vi "Periodic Tasks.vi"(8 "error in (no error)":errorcluster) -> ()   [LabVIEW 2017]
doc: "This VI runs in parallel to other tasks. It can contain as many user-defined periodic loops as you need. These can carry out PID or other sorts of timed response."
uses:
  Robot Global Data.vi
  <vilib>/Rock Robotics/WPI/Utilities/WPI_GetSetVariantRefNum.vi
  <vilib>/addons/control/pid/pid.llb/PID (DBL).vi
  <vilib>/Rock Robotics/Network Tables/NT Read Number.vi
  <vilib>/Rock Robotics/WPI/RobotDrive/WPI_RobotDriveArcadeDrive_Standard(NoSaturation).vi
  <vilib>/Rock Robotics/Network Tables/NT Write Number.vi
  <vilib>/addons/control/pid/NI_PID_pid.lvlib
  <vilib>/Analysis/NI_AALPro.lvlib
  <vilib>/Analysis/coordinate.llb/2D Cartesian Coordinate Shift (Scalar).vi
  <vilib>/Rock Robotics/Network Tables/NT Read String.vi
  <vilib>/Analysis/coordinate.llb/2D Cartesian Coordinate Shift (Array).vi
  <vilib>/Analysis/coordinate.llb/2D Cartesian Coordinate Rotation (Scalar).vi
panel:
  out "Waveform Chart":dbl(graph)
  out "CDF Arm Down":bool
  out "error out (no error)":errorcluster
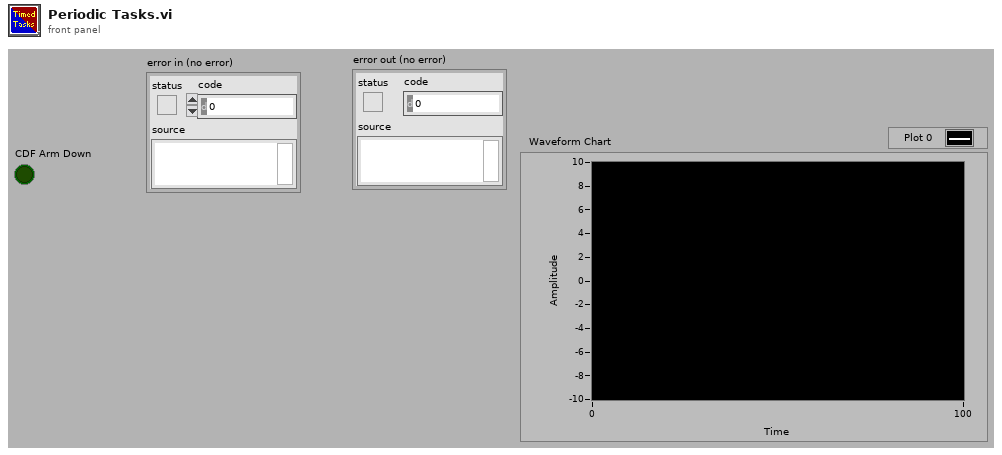
[diagram p1: front panel]
types:
  T1 = cluster{"theta":dbl, "x":dbl, "y":dbl, "xServo":dbl, "yServo":dbl}
  T2 = typedef "WPI_PotentiometerDevRef.ctl" = cluster{"DevStatus":errorcluster, "Analog Channel":T3, "Invert Output":bool}
  T3 = typedef "FPGA_AIChannel.ctl" = enum8{"AI 0", "AI 1", "AI 2", "AI 3", "AI MXP 0", "AI MXP 1", "AI MXP 2", "AI MXP 3", "Invalid"}
  T4 = typedef "WPI_ServoDeviceRef.ctl" = cluster{"DeviceStatus":errorcluster, "PWM Channel":T5, "DeadBand":T6}
  T5 = typedef "FPGA_DIOPWMChannel.ctl" = enum8{"PWM 0", "PWM 1", "PWM 2", "PWM 3", "PWM 4", "PWM 5", "PWM 6", "PWM 7", "PWM 8", "PWM 9", "PWM MXP 0", "PWM MXP 1", "PWM MXP 2", "PWM MXP 3", "PWM MXP 4", "PWM MXP 5", "PWM MXP 6", "PWM MXP 7", "PWM MXP 8", "PWM MXP 9", "Invalid"}
  T6 = typedef "WPI_PWMDeadband.ctl" = cluster{"Name":string, "maxPositivePwm":i32, "minPositivePwm":i32, "centerPwm":i32, "maxNegativePwm":i32, "minNegativePwm":i32, "angularRange":u16}
  T7 = typedef "WPI_GyroDevRef.ctl" = cluster{"DevStatus":errorcluster, "Analog Channel":T3, "Gain (VoltsPerDegree/Second)":dbl, "Gyro Type":enum16{"Analog", "XRS450"}, "Handle":i32, "SPI Bus":T8, "Device Found":bool, "Sample Rate":dbl, "Calibrate On Open":bool, "Offset":dbl}
  T8 = typedef "spi_bus.ctl" = enum16{"SPI On-Board, CS0", "SPI On-Board, CS1", "SPI On-Board, CS2", "SPI On-Board, CS3", "SPI MXP", "Invalid"}
  T9 = cluster{"theta":dbl, "x":dbl, "y":dbl, "xServo":dbl, "yServo":dbl}[]
  T10 = typedef "WPI_RobotDriveDevRef.ctl" = cluster{"DevStatus":errorcluster, "Motors[]":T11[], "Square Inputs":bool, "Max Output":dbl}
  T11 = typedef "WPI_MotorControlDeviceRef.ctl" = cluster{"DeviceStatus":errorcluster, "Type":T12, "PWM":cluster{"PWM Channel":T5, "DeadBand":T6}, "CAN":cluster{"Device Number":u8, "SetOutput VI Ref":variant, "GetOutput VI Ref":variant, "Enable VI Ref":variant, "Disable VI Ref":variant, "Data":variant}, "Invert":bool, "DIO PWM":cluster{"PWM \"Enable\" Channel":T5, "DIOChannel":T13, "PWM Rate":dbl}}
  T12 = typedef "WPI_MotorControlType.ctl" = enum16{"PWM", "CAN", "DIO PWM"}
  T13 = typedef "FPGA_DIOChannel.ctl" = enum8{"DIO 0", "DIO 1", "DIO 2", "DIO 3", "DIO 4", "DIO 5", "DIO 6", "DIO 7", "DIO 8", "DIO 9", "DIO MXP 0", "DIO MXP 1", "DIO MXP 2", "DIO MXP 3", "DIO MXP 4", "DIO MXP 5", "DIO MXP 6", "DIO MXP 7", "DIO MXP 8", "DIO MXP 9", "DIO MXP 10", "DIO MXP 11", "DIO MXP 12", "DIO MXP 13", "DIO MXP 14", "DIO MXP 15", "SPI Port CS1", "SPI Port CS2", "SPI Port CS3", "SPI Port MISO", "SPI Port MOSI", "Invalid"}
  T14 = cluster{"proportional gain (Kc)":dbl, "integral time (Ti, min)":dbl, "derivative time (Td, min)":dbl}
  T15 = typedef "WPI_AccelerometerDevRef.ctl" = cluster{"DevStatus":errorcluster, "Scaling":T16, "Analog Channels":T17, "I2C Bus":T18, "SPI Bus":T8, "Accel Range":T19, "ADXL Axes":T20, "Handle":i32, "Device Address":u8, "Accel Type":enum16{"Analog", "ADXL345 I2C", "ADXL345 SPI", "Internal", "ADXL362 SPI"}}
  T16 = typedef "WPI_AccelerometerScaling.ctl" = cluster{"Gain (VoltsPerG)":dbl, "Center Voltage":dbl}
  T17 = typedef "WPI_AccelerometerAnalogChannels.ctl" = cluster{"X-Axis":T3, "Y-Axis":T3, "Z-Axis":T3}
  T18 = typedef "i2c_bus.ctl" = enum16{"I2C On-Board", "I2C MXP", "Invalid"}
  T19 = typedef "ADXL345 Range.ctl" = u8
  T20 = typedef "WPI_AccelerometerADXL345 Axes.ctl" = cluster{"X-Axis":bool, "Y-Axis":bool, "Z-Axis":bool}
  T21 = cluster{"X-Axis":dbl, "Y-Axis":dbl, "Z-Axis":dbl}
  T22 = enum16{"open", "replace", "create", "open or create", "replace or create", "replace or create with confirmation"}
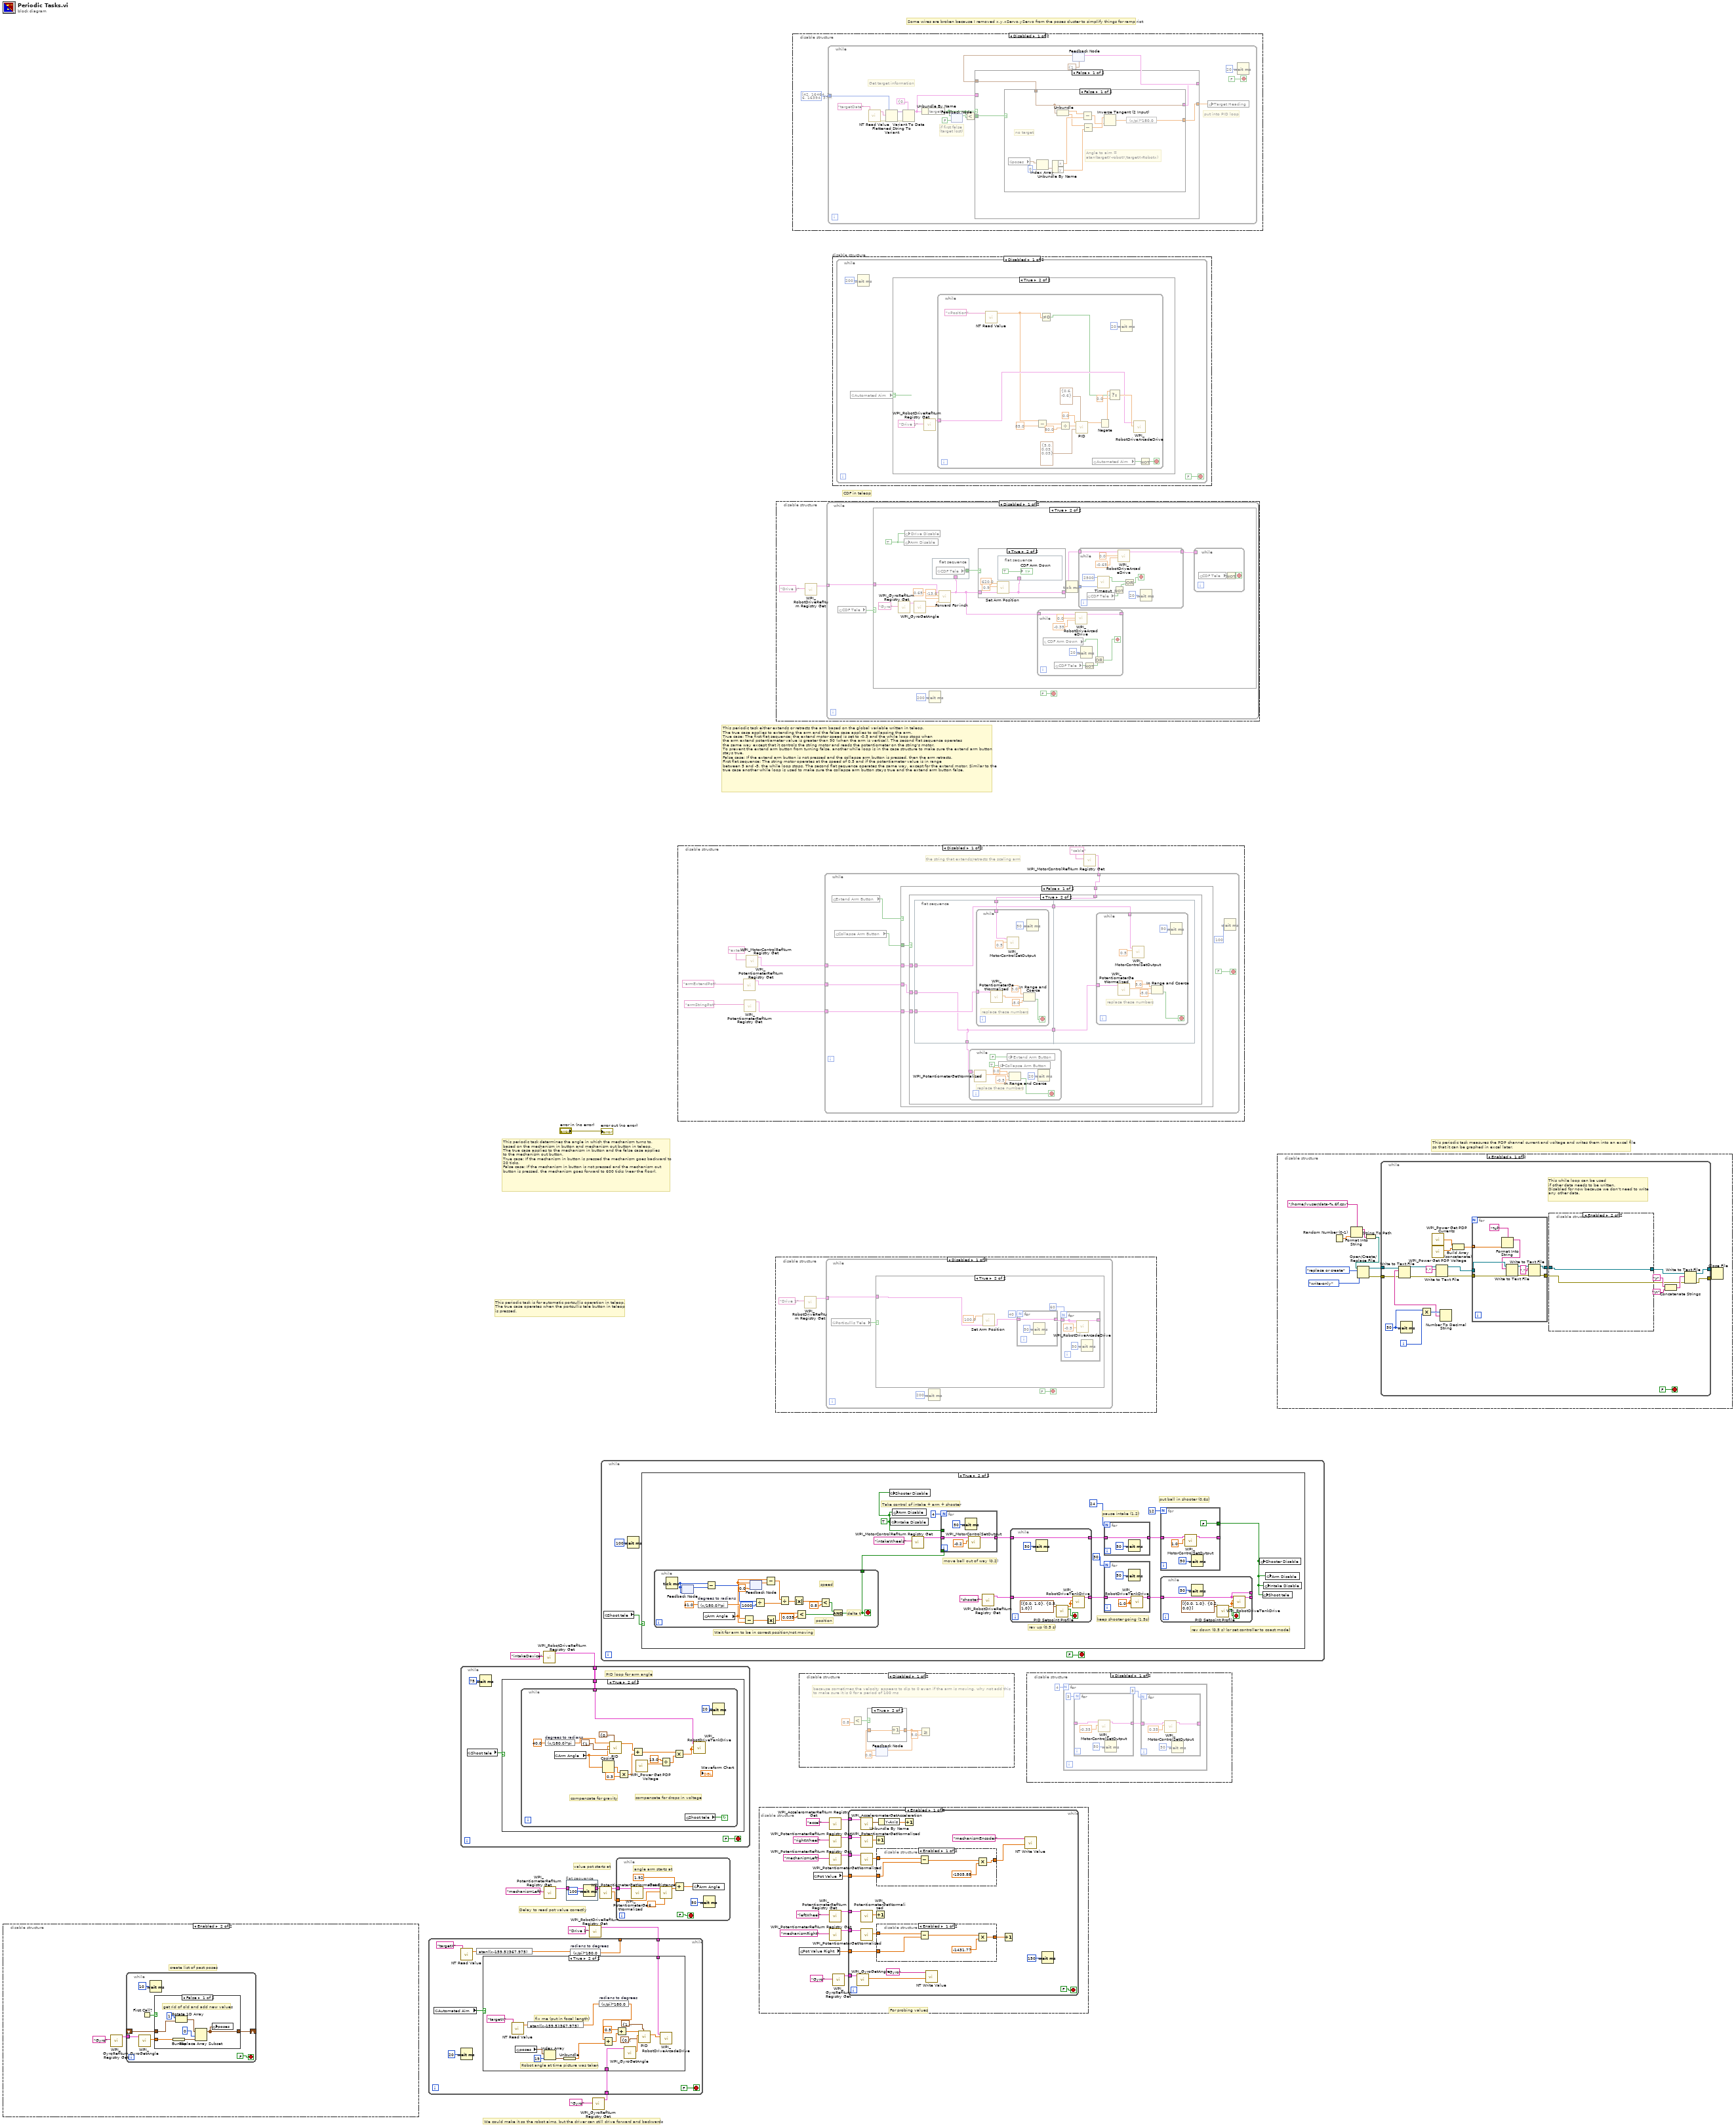
[diagram p0: block diagram]
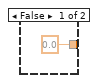
[diagram p4: hidden frame]
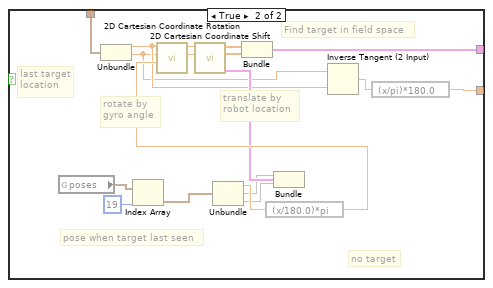
[diagram p8: hidden frame]
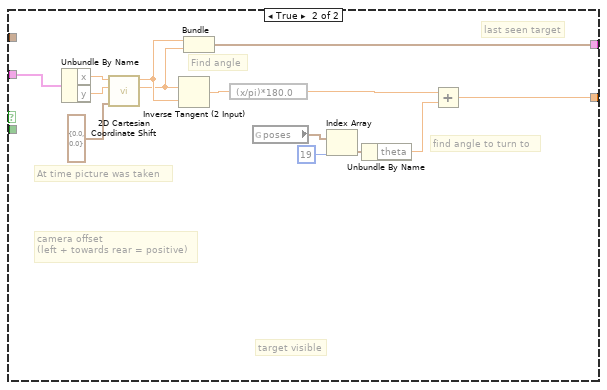
[diagram p9: hidden frame]
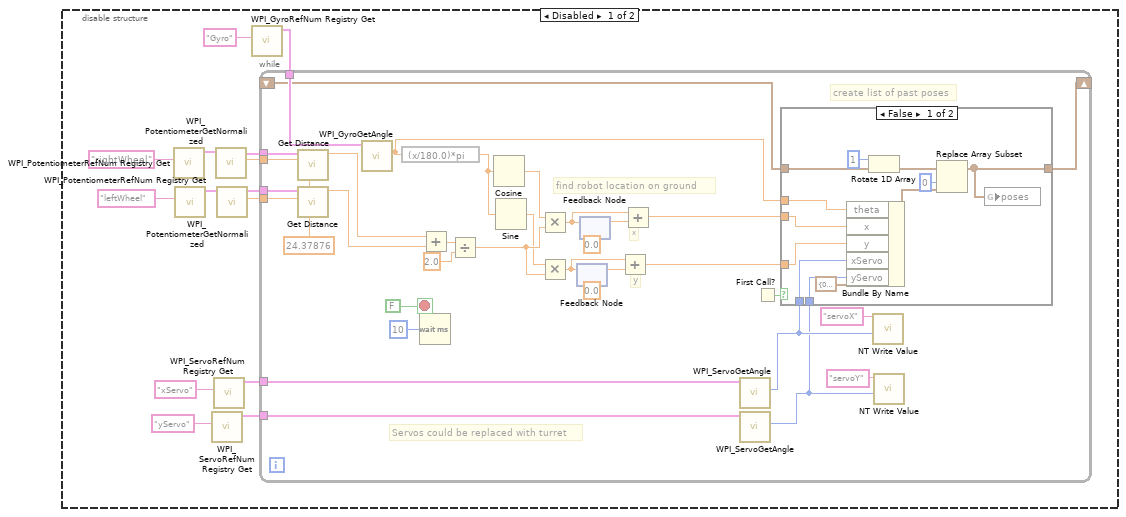
[diagram p11: hidden frame]
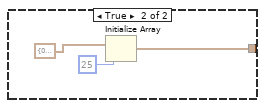
[diagram p12: hidden frame]
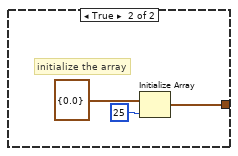
[diagram p13: hidden frame]
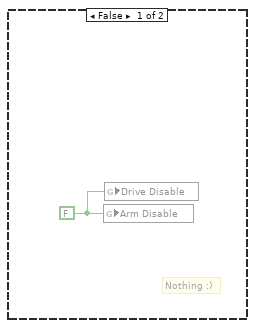
[diagram p16: hidden frame]
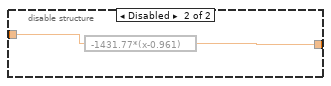
[diagram p19: hidden frame]
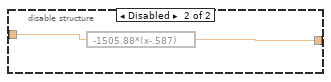
[diagram p20: hidden frame]
diagram:
  # "We could make it so the robot aims, but the driver can still drive forward and backwards"
  # "Delay to read pot value correctly"
  # "Some wires are broken because I removed x,y,xServo,yServo from the poses cluster to simplify things for ramp riot"
  # "value pot starts at"
  # "CDF in teleop"
  # "This periodic task either extends or retracts the arm based on the global variable written in teleop.\nThe true case applies to extending the arm and the false case applies to collapsing the arm. \nTrue case: The first flat sequence: the extend motor speed is set to -0.5 and the while loop stops when\nthe arm extend potentiameter value is greater than 90 (when the arm is vertical). The second flat sequence operates\nthe same way except that it controls the string motor and reads the potentiometer on the string's motor. \nTo prevent the extend arm button from turning false, another while loop is in the case structure to make sure the extend arm button \nstays true. \nFalse case: If the extend arm button is not pressed and the collapse arm button is pressed, then the arm retracts.\nFirst flat sequence: The string motor operates at the speed of 0.5 and if the potentiameter value is in range \nbetween 5 and -5, the while loop stops. The second flat sequence operates the same way, except for the extend motor. Similar to the \ntrue case another while loop is used to make sure the collapse arm button stays true and the extend arm button false."
  # "This periodic task measures the PDP channel current and voltage and writes them into an excel file \nso that it can be graphed in excel later."
  # "This periodic task is for automatic portcullis operation in teleop. \nThe true case operates when the portcullis tele button in teleop \nis pressed."
  # "This periodic task determines the angle in which the mechanism turns to, \nbased on the mechanism in button and mechanism out button in teleop.\nThe true case applies to the mechanism in button and the false case applies\nto the mechanism out button. \nTrue case: If the mechanism in button is pressed the mechanism goes backward to\n20 ticks. \nFalse case: If the mechanism in button is not pressed and the mechanism out\nbutton is pressed, the mechanism goes forward to 600 ticks (near the floor)."
  n1 = disable-structure shown="Enabled" {
    frame Disabled {
      n2 = call <vilib>:"WPI_PotentiometerRefNum Registry Get.vi"("refnum name"="rightWheel") -> ("PotDevRef"=w26:T2)  [unwired: 9 in, 1 out]
      n3 = call <vilib>:"WPI_PotentiometerRefNum Registry Get.vi"("refnum name"="leftWheel") -> ("PotDevRef"=w24:T2)  [unwired: 9 in, 1 out]
      n4 = call <vilib>:"WPI_ServoRefNum Registry Get.vi"("refnum name"="yServo") -> ("ServoDeviceRef"=w13:T4)  [unwired: 9 in, 1 out]
      n5 = call <vilib>:"WPI_ServoRefNum Registry Get.vi"("refnum name"="xServo") -> ("ServoDeviceRef"=w14:T4)  [unwired: 9 in, 1 out]
      n6 = call <vilib>:"WPI_PotentiometerGetNormalized.vi"("PotDevRef"=w26) -> ("Normalized Value"=w18:dbl, "PotDevRef"=w21:T2)  [unwired: 8 in, 1 out]
      n7 = call <vilib>:"WPI_PotentiometerGetNormalized.vi"("PotDevRef"=w24) -> ("Normalized Value"=w19:dbl, "PotDevRef"=w20:T2)  [unwired: 8 in, 1 out]
      n8 = call <vilib>:"WPI_GyroRefNum Registry Get.vi"("refnum name"="Gyro") -> ("GyroDevRef"=w17:T7)  [unwired: 9 in, 1 out]
      n9 = while {
        tunnel: w21 -> [w59]
        tunnel: w20 -> [w58]
        tunnel: w19 -> [w57]
        tunnel: w18 -> [w56]
        tunnel: w17 -> [w39]
        shift-right: [w35] -> _
        shift-left: _ -> [w34]
        tunnel: w14 -> [w30]
        tunnel: w13 -> [w29]
        stop <- FALSE stop-if-true
        w55 = 24.37876 ("distance/rotation")
        # "Servos could be replaced with turret"
        # "create list of past poses"
        # "find robot location on ground"
        # "y"
        # "x"
        n10 = call "Get Distance.vi"("distance/rotation"=w55, "Starting value"=w56, "PotDevRef"=w59) -> ("Distance"=w41:dbl)  [unwired: 8 in]
        n11 = call "Get Distance.vi"("distance/rotation"=w55, "Starting value"=w57, "PotDevRef"=w58) -> ("Distance"=w40:dbl)  [unwired: 8 in]
        n12 = call <vilib>:"WPI_GyroGetAngle.vi"("GyroDevRef"=w39) -> ("Angle"=w33:dbl)  [unwired: 6 in, 4 out]
        n13 = expression code="(x/180.0)*pi" ("degrees to radians")(w33) -> (w50:dbl)
        n14 = Wait (ms)(milliseconds to wait=u32 10) -> ()  [unwired: 1 out]
        n15 = Add(x=w41, y=w40) -> (x+y=w53:dbl)
        n16 = Divide(x=w53, y=2.0) -> (x/y=w49:dbl)
        n17 = Cosine(x=w50) -> (cos(x)=w51:dbl)
        n18 = Sine(x=w50) -> (sin(x)=w48:dbl)
        n19 = Multiply(x=w51, y=w49) -> (x*y=w46:dbl)
        n20 = Multiply(x=w48, y=w49) -> (x*y=w42:dbl)
        n21 = feedback #1(0.0) -> (w43:dbl)
        n22 = feedback-in #1(w42) -> ()
        n23 = feedback #2(0.0) -> (w47:dbl)
        n24 = feedback-in #2(w46) -> ()
        n25 = Add(x=w42, y=w43) -> (x+y=w32:dbl)
        n26 = Add(x=w46, y=w47) -> (x+y=w31:dbl)
        n27 = call <vilib>:"WPI_ServoGetAngle.vi"("ServoDeviceRef"=w30) -> ("Angle"=w28:u16)  [unwired: 7 in, 2 out]
        n28 = call <vilib>:"WPI_ServoGetAngle.vi"("ServoDeviceRef"=w29) -> ("Angle"=w27:u16)  [unwired: 7 in, 2 out]
        n29 = First Call?() -> (First Call?: T/F=w38:bool)
        n30 = case shown="False" w38 {
          tunnel: [w61 w74] -> w35
          tunnel: w34 -> [w72 _]
          tunnel: w33 -> [w68 _]
          tunnel: w31 -> [w64 _]
          tunnel: w32 -> [w65 _]
          tunnel: w28 -> [w63 _]
          tunnel: w27 -> [w62 _]
          frame False {
            n31 = Bundle By Name(cluster=T1 {"theta"=0.0, "x"=0.0, "y"=0.0, "xServo"=0.0, "yServo"=0.0}, "theta"=w68, "x"=w64, "y"=w65, "xServo"=w63, "yServo"=w62) -> (w66:T1)
            n32 = Rotate 1D Array(1:w72, 2:1 ("n")) -> (0:w70:T9)
            n33 = Replace Array Subset(array=w70, new element=w66, index=0) -> (w61:T9)
            n34 = global write "Robot Global Data.vi" "poses"(w61) -> ()
          }
          frame True {
            n35 = Initialize Array(T1 {"theta"=0.0, "x"=0.0, "y"=0.0, "xServo"=0.0, "yServo"=0.0}, 25 ("dimension size")) -> (w74:T9)
          }
        }
        n36 = call-poly <vilib>:"NT Write Value.vi"("Numeric"=w28, "Name"="servoX") -> ()  [unwired: 9 in, 1 out]
        n37 = call-poly <vilib>:"NT Write Value.vi"("Numeric"=w27, "Name"="servoY") -> ()  [unwired: 9 in, 1 out]
      }
    }
    frame Enabled {
      # "create list of past poses"
      n38 = call <vilib>:"WPI_GyroRefNum Registry Get.vi"("refnum name"="Gyro") -> ("GyroDevRef"=w76:T7)  [unwired: 9 in, 1 out]
      n39 = while {
        tunnel: w76 -> [w82]
        shift-right: [w80] -> _
        shift-left: _ -> [w79]
        stop <- FALSE stop-if-true
        n40 = call <vilib>:"WPI_GyroGetAngle.vi"("GyroDevRef"=w82) -> ("Angle"=w78:dbl)  [unwired: 6 in, 4 out]
        n41 = First Call?() -> (First Call?: T/F=w81:bool)
        n42 = Wait (ms)(milliseconds to wait=u32 10) -> ()  [unwired: 1 out]
        n43 = case shown="False" w81 {
          tunnel: [w87 w93] -> w80
          tunnel: w79 -> [w91 _]
          tunnel: w78 -> [w86 _]
          frame False {
            # "get rid of old and add new values"
            n44 = Bundle("Angle"=w86) -> (w85:cluster{"Angle":dbl})  [unwired: 1 in]
            n45 = Rotate 1D Array(1:w91, 2:1 ("n")) -> (0:w89:cluster{"theta":dbl}[])
            n46 = Replace Array Subset(array=w89, new element=w85, index=0) -> (w87:cluster{"theta":dbl}[])
            n47 = global write "Robot Global Data.vi" "poses"(w87) -> ()
          }
          frame True {
            # "initialize the array"
            n48 = Initialize Array(cluster{"theta":dbl} {"theta"=0.0}, 25 ("dimension size")) -> (w93:cluster{"theta":dbl}[])
          }
        }
      }
    }
  }
  n49 = call <vilib>:"WPI_RobotDriveRefNum Registry Get.vi"("refnum name"="intakeDevice") -> ("RobotDriveDevRef"=w5:T10)  [unwired: 9 in, 1 out]
  n50 = while {
    tunnel: w5 -> [w95]
    stop <- FALSE stop-if-true
    # "PID loop for arm angle"
    n51 = global read "Robot Global Data.vi" "Shoot tele"() -> (w98:bool)
    n52 = Wait (ms)(milliseconds to wait=u32 75) -> ()  [unwired: 1 out]
    n53 = case shown="True" w98 {
      tunnel: w95 -> [_ w99]
      frame False {
      }
      frame True {
        n54 = while {
          tunnel: w99 -> [w113]
          stop <- w115 continue-if-true
          # "compensate for drops in voltage"
          # "compensate for gravity"
          n55 = expression code="(x/180.0)*pi" "degrees to radians"(40.0 ("angle B 2")) -> (w110:dbl)
          n56 = global read "Robot Global Data.vi" "Arm Angle"() -> (w101:dbl)
          n57 = Cosine(x=w101) -> (cos(x)=w108:dbl)
          n58 = call-poly <vilib>:"PID.vi"("output range"=cluster{"output high":dbl, "output low":dbl} {"output high"=0.7, "output low"=-0.7}, "PID gains"=T14 {"proportional gain (Kc)"=1.1, "integral time (Ti, min)"=0.008, "derivative time (Td, min)"=0.0001} ("PID arm gains"), "process variable"=w101, "setpoint"=w110) -> ("output"=w107:dbl)  [unwired: 6 in, 1 out]
          n59 = Multiply(x=w108, y=0.3) -> (x*y=w106:dbl)
          n60 = Add(x=w107, y=w106) -> (x+y=w103:dbl)
          n61 = call <vilib>:"WPI_Power Get PDP Voltage.vi"() -> ("voltage (V)"=w104:dbl)  [unwired: 14 in, 1 out]
          n62 = Divide(x=13.0, y=w104) -> (x/y=w100:dbl)
          n63 = Multiply(x=w103, y=w100) -> (x*y=w102:dbl)
          n64 = global read "Robot Global Data.vi" "Shoot tele"() -> (w115:bool)
          n65 = call <vilib>:"WPI_RobotDriveTankDrive.vi"("Right axis value"=w102, "Left axis value"=w102, "RobotDriveDevRef"=w113) -> ()  [unwired: 6 in, 3 out]
          n66 = Wait (ms)(milliseconds to wait=u32 20) -> ()  [unwired: 1 out]
        }
      }
    }
  }
  n67 = call <vilib>:"WPI_PotentiometerRefNum Registry Get.vi"("refnum name"="mechanismLeft") -> ("PotDevRef"=w8:T2)  [unwired: 9 in, 1 out]
  n68 = flat-sequence {
    tunnel: w8 -> [w118]
    tunnel: [w118] -> w7
    frame #0 {
      n69 = Wait (ms)(milliseconds to wait=u32 100) -> ()  [unwired: 1 out]
    }
  }
  n70 = call <vilib>:"WPI_RobotDriveRefNum Registry Get.vi"("refnum name"="Drive 1") -> ("RobotDriveDevRef"=w3:T10)  [unwired: 9 in, 1 out]
  n71 = call <vilib>:"WPI_GyroRefNum Registry Get.vi"("refnum name"="Gyro") -> ("GyroDevRef"=w1:T7)  [unwired: 9 in, 1 out]
  n72 = while {
    tunnel: w3 -> [w124]
    tunnel: w1 -> [w123]
    tunnel: [w119] -> _
    stop <- FALSE stop-if-true
    n73 = global read "Robot Global Data.vi" "Automated Aim"() -> (w125:bool)
    n74 = call-poly <vilib>:"NT Read Value.vi"("Name"="targetX") -> ("Numeric"=w122:dbl)  [unwired: 9 in, 1 out]
    n75 = Wait (ms)(milliseconds to wait=u32 20) -> ()  [unwired: 1 out]
    n76 = expression code="atan((x-159.5)/367.975)"(w122) -> (w120:dbl)
    n77 = case shown="True" w125 {
      tunnel: w124 -> [_ w138]
      tunnel: w123 -> [_ w137]
      frame False {
      }
      frame True {
        # "fix me (put in focal length)"
        # "Robot angle at time picture was taken"
        n78 = call-poly <vilib>:"NT Read Value.vi"("Name"="targetX") -> ("Numeric"=w143:dbl)  [unwired: 9 in, 1 out]
        n79 = global read "Robot Global Data.vi" "poses"() -> (w142:cluster{"theta":dbl}[])
        n80 = expression code="atan((x-159.5)/367.975)"(w143) -> (w135:dbl)
        n81 = Index Array(array=w142, index=19) -> (element=w140:cluster{"theta":dbl})
        n82 = Unbundle(w140) -> ("theta"=w139:dbl)
        n83 = expression code="(x/pi)*180.0" "radians to degrees"(w135) -> (w134:dbl)
        n84 = Add(x=w134, y=w139) -> (x+y=w130:dbl)
        n85 = Add(x=0.5, y=w130) -> (x+y=w128:dbl)
        n86 = call <vilib>:"WPI_GyroGetAngle.vi"("GyroDevRef"=w137) -> ("Angle"=w136:dbl)  [unwired: 6 in, 4 out]
        n87 = call-poly <vilib>:"PID.vi"("output range"=cluster{"output high":dbl, "output low":dbl} {"output high"=1.0, "output low"=-1.0}, "PID gains"=T14 {"proportional gain (Kc)"=0.07, "integral time (Ti, min)"=0.004, "derivative time (Td, min)"=1e-05} ("PID turn angle gains"), "process variable"=w136, "setpoint"=w128) -> ("output"=w133:dbl)  [unwired: 6 in, 1 out]
        n88 = call-poly <vilib>:"WPI_RobotDriveArcadeDrive.vi"("X axis value"=w133, "RobotDriveDevRef"=w138) -> ()  [unwired: 7 in, 3 out]
      }
    }
    n89 = expression code="(x/pi)*180.0" "radians to degrees"(w120) -> (w119:dbl)
  }
  n90 = call <vilib>:"WPI_PotentiometerGetNormalized.vi"("PotDevRef"=w7) -> ("Normalized Value"=w9:dbl, "PotDevRef"=w10:T2)  [unwired: 8 in, 1 out]
  n91 = while {
    stop <- FALSE stop-if-true
    n92 = global read "Robot Global Data.vi" "Shoot tele"() -> (w145:bool)
    n93 = Wait (ms)(milliseconds to wait=u32 100) -> ()  [unwired: 1 out]
    n94 = case shown="True" w145 {
      frame False {
      }
      frame True {
        w149 = TRUE ("Intake Disable")
        # "Wait for arm to be in correct position/not moving"
        # "Take control of intake + arm + shooter"
        # "put ball in shooter (0.6s)"
        # "pause intake (1.2)"
        # "rev down (0.5 s) (or set controller to coast mode)"
        # "keep shooter going (1.5s)"
        # "rev up (0.5 s)"
        # "move ball out of way (0.2)"
        n95 = while {
          tunnel: [w164] -> w156
          stop <- w164 stop-if-true
          # "position"
          # "speed"
          # "delta t"
          n96 = Tick Count (ms)() -> (millisecond timer value=w177:u32)
          n97 = feedback #3(w177) -> (w176:u32)
          n98 = feedback-in #3(w177) -> ()
          n99 = expression code="(x/180.0)*pi" "degrees to radians"(41.0 ("angle B 2")) -> (w171:dbl)
          n100 = global read "Robot Global Data.vi" "Arm Angle"() -> (w170:dbl)
          n101 = Subtract(x=w177, y=w176) -> (x-y=w178:u32)
          n102 = Subtract(x=w171, y=w170) -> (x-y=w166:dbl)
          n103 = feedback #4(0.0 ("Arm Angle")) -> (w180:dbl)
          n104 = feedback-in #4(w170) -> ()
          n105 = Divide(x=w178, y=u32 1000) -> (x/y=w183:dbl)
          n106 = Subtract(x=w170, y=w180) -> (x-y=w182:dbl)
          n107 = Absolute Value(x=w166) -> (abs(x)=w165:dbl)
          n108 = Divide(x=w182, y=w183) -> (x/y=w175:dbl)
          n109 = Absolute Value(x=w175) -> (abs(x)=w172:dbl)
          n110 = Less?(x=w165, y=0.035) -> (x < y?=w168:bool)
          n111 = Less?(x=w172, y=0.8) -> (x < y?=w173:bool)
          n112 = And(x=w173, y=w168) -> (x .and. y?=w164:bool)
        }
        n113 = global write "Robot Global Data.vi" "Shooter Disable"(w149) -> ()
        n114 = global write "Robot Global Data.vi" "Intake Disable"(w149) -> ()
        n115 = global write "Robot Global Data.vi" "Arm Disable"(w149) -> ()
        n116 = call <vilib>:"WPI_MotorControlRefNum Registry Get.vi"("refnum name"="intakeWheels") -> ("MotorControlDevRef"=w154:T11)  [unwired: 9 in, 1 out]
        n117 = for {
          N: 4 -> [_]
          tunnel: w154 -> [w201]
          tunnel: [w203] -> w152
          tunnel: w149 -> [_]
          tunnel: w156 -> [_]
          n118 = Wait (ms)(milliseconds to wait=u32 50) -> ()  [unwired: 1 out]
          n119 = call <vilib>:"WPI_MotorControlSetOutput.vi"("Output"=-0.2 ("Left axis value"), "MotorControlDevRef"=w201) -> ("MotorControlDevRef"=w203:T11)  [unwired: 7 in, 2 out]
        }
        n120 = call <vilib>:"WPI_RobotDriveRefNum Registry Get.vi"("refnum name"="shooter") -> ("RobotDriveDevRef"=w150:T10)  [unwired: 9 in, 1 out]
        n121 = while {
          tunnel: w150 -> [w209]
          tunnel: [w208] -> w162
          tunnel: [w205] -> w153
          tunnel: w152 -> [w205]
          stop <- w211 stop-if-true
          n122 = Wait (ms)(milliseconds to wait=u32 50) -> ()  [unwired: 1 out]
          n123 = call <vilib>:"PID Setpoint Profile.vi"("setpoint profile"=cluster{"time (s)":dbl, "setpoint":dbl}[] [{"time (s)"=0.0, "setpoint"=1.0}, {"time (s)"=0.5, "setpoint"=1.0}]) -> ("profile complete?"=w211:bool, "setpoint"=w210:dbl)  [unwired: 5 in, 2 out]
          n124 = call <vilib>:"WPI_RobotDriveTankDrive.vi"("Right axis value"=w210, "Left axis value"=w210, "RobotDriveDevRef"=w209) -> ("RobotDriveDevRef"=w208:T10)  [unwired: 6 in, 2 out]
        }
        n125 = for {
          N: 24 -> [_]
          tunnel: [w195] -> w159
          tunnel: w153 -> [w195]
          n126 = Wait (ms)(milliseconds to wait=u32 50) -> ()  [unwired: 1 out]
        }
        n127 = for {
          N: 30 -> [_]
          tunnel: w162 -> [w199]
          tunnel: [w197] -> w157
          w200 = -1.0 ("Left axis value")
          n128 = Wait (ms)(milliseconds to wait=u32 50) -> ()  [unwired: 1 out]
          n129 = call <vilib>:"WPI_RobotDriveTankDrive.vi"("Right axis value"=w200, "Left axis value"=w200, "RobotDriveDevRef"=w199) -> ("RobotDriveDevRef"=w197:T10)  [unwired: 6 in, 2 out]
        }
        n130 = for {
          N: 12 -> [_]
          tunnel: w159 -> [w191]
          tunnel: [w192] -> _
          tunnel: [FALSE ("Shoot tele")] -> w148
          n131 = call <vilib>:"WPI_MotorControlSetOutput.vi"("Output"=1.0 ("Left axis value"), "MotorControlDevRef"=w191) -> ("MotorControlDevRef"=w192:T11)  [unwired: 7 in, 2 out]
          n132 = Wait (ms)(milliseconds to wait=u32 50) -> ()  [unwired: 1 out]
        }
        n133 = while {
          tunnel: [w184] -> _
          tunnel: [w186] -> _
          tunnel: w157 -> [w184]
          stop <- w188 stop-if-true
          n134 = Wait (ms)(milliseconds to wait=u32 50) -> ()  [unwired: 1 out]
          n135 = call <vilib>:"PID Setpoint Profile.vi"("setpoint profile"=cluster{"time (s)":dbl, "setpoint":dbl}[] [{"time (s)"=0.0, "setpoint"=1.0}, {"time (s)"=0.2, "setpoint"=0.0}]) -> ("profile complete?"=w188:bool, "setpoint"=w187:dbl)  [unwired: 5 in, 2 out]
          n136 = call <vilib>:"WPI_RobotDriveTankDrive.vi"("Right axis value"=w187, "Left axis value"=w187, "RobotDriveDevRef"=w184) -> ("RobotDriveDevRef"=w186:T10)  [unwired: 6 in, 2 out]
        }
        n137 = global write "Robot Global Data.vi" "Shooter Disable"(w148) -> ()
        n138 = global write "Robot Global Data.vi" "Shoot tele"(w148) -> ()
        n139 = global write "Robot Global Data.vi" "Intake Disable"(w148) -> ()
        n140 = global write "Robot Global Data.vi" "Arm Disable"(w148) -> ()
      }
    }
  }
  n141 = while {
    tunnel: w10 -> [w220]
    tunnel: w9 -> [w215]
    stop <- FALSE stop-if-true
    # "angle arm starts at"
    n142 = call <vilib>:"WPI_PotentiometerGetNormalized.vi"("PotDevRef"=w220) -> ("PotDevRef"=w218:T2)  [unwired: 8 in, 2 out]
    n143 = call "Get Distance.vi"("distance/rotation"=6.283185307179586, "Starting value"=w215, "PotDevRef"=w218) -> ("Distance"=w214:dbl)  [unwired: 8 in]
    n144 = Add(x=1.92 ("Starting value"), y=w214) -> (x+y=w213:dbl)
    n145 = global write "Robot Global Data.vi" "Arm Angle"(w213) -> ()
    n146 = Wait (ms)(milliseconds to wait=u32 50) -> ()  [unwired: 1 out]
  }
  n147 = disable-structure shown="Disabled" {
    frame Disabled {
      # "the string that extends/retracts the scaling arm"
      n148 = call <vilib>:"WPI_PotentiometerRefNum Registry Get.vi"("refnum name"="armExtendPot") -> ("PotDevRef"=w224:T2)  [unwired: 9 in, 1 out]
      n149 = call <vilib>:"WPI_PotentiometerRefNum Registry Get.vi"("refnum name"="armStringPot") -> ("PotDevRef"=w223:T2)  [unwired: 9 in, 1 out]
      n150 = call <vilib>:"WPI_MotorControlRefNum Registry Get.vi"("refnum name"="extend") -> ("MotorControlDevRef"=w222:T11)  [unwired: 9 in, 1 out]
      n151 = call <vilib>:"WPI_MotorControlRefNum Registry Get.vi"("refnum name"="cable") -> ("MotorControlDevRef"=w221:T11)  [unwired: 9 in, 1 out]
      n152 = while {
        tunnel: w224 -> [w235]
        tunnel: w223 -> [w234]
        tunnel: w222 -> [w232]
        tunnel: w221 -> [w231]
        stop <- FALSE stop-if-true
        n153 = global read "Robot Global Data.vi" "Extend Arm Button"() -> (w230:bool)
        n154 = global read "Robot Global Data.vi" "Collapse Arm Button"() -> (w229:bool)
        n155 = case shown="False" w230 {
          tunnel: w229 -> [w241 _]
          tunnel: w235 -> [w240 w284]
          tunnel: w234 -> [w239 w282]
          tunnel: w232 -> [w237 w281]
          tunnel: w231 -> [w238 w280]
          frame False {
            n156 = case shown="True" w241 {
              tunnel: w240 -> [_ w248]
              tunnel: w239 -> [_ w247]
              tunnel: w238 -> [_ w246]
              tunnel: w237 -> [_ w244]
              frame False {
                # "Nothing :)"
              }
              frame True {
                n157 = flat-sequence {
                  tunnel: w248 -> [w257]
                  tunnel: w247 -> [w258]
                  tunnel: w246 -> [w260]
                  tunnel: [w259] -> w245
                  tunnel: w244 -> [w259]
                  tunnel: [w257] -> w243
                  tunnel: [w257] -> w242
                  tunnel: w245 -> [w270]
                  tunnel: w243 -> [w269]
                  frame #0 {
                    n158 = while {
                      tunnel: w260 -> [w267]
                      tunnel: w258 -> [w266]
                      stop <- w261 stop-if-true
                      # "replace these numbers"
                      n159 = call <vilib>:"WPI_PotentiometerGetNormalized.vi"("PotDevRef"=w266) -> ("Normalized Value"=w264:dbl)  [unwired: 8 in, 2 out]
                      n160 = call <vilib>:"WPI_MotorControlSetOutput.vi"("Output"=0.5, "MotorControlDevRef"=w267) -> ()  [unwired: 7 in, 3 out]
                      n161 = In Range and Coerce(upper limit=5.0, x=w264, lower limit=-5.0) -> (In Range?=w261:bool)  [unwired: 1 out]
                      n162 = Wait (ms)(milliseconds to wait=u32 50) -> ()  [unwired: 1 out]
                    }
                  }
                  frame #1 {
                    n163 = while {
                      tunnel: w270 -> [w277]
                      tunnel: w269 -> [w276]
                      stop <- w274 stop-if-true
                      # "replace these numbers"
                      n164 = call <vilib>:"WPI_PotentiometerGetNormalized.vi"("PotDevRef"=w276) -> ("Normalized Value"=w272:dbl)  [unwired: 8 in, 2 out]
                      n165 = call <vilib>:"WPI_MotorControlSetOutput.vi"("Output"=0.5, "MotorControlDevRef"=w277) -> ()  [unwired: 7 in, 3 out]
                      n166 = In Range and Coerce(upper limit=5.0 ("y"), x=w272, lower limit=-5.0) -> (In Range?=w274:bool)  [unwired: 1 out]
                      n167 = Wait (ms)(milliseconds to wait=u32 50) -> ()  [unwired: 1 out]
                    }
                  }
                }
                n168 = while {
                  tunnel: w242 -> [w256]
                  stop <- w249 stop-if-true
                  # "Extend"
                  # "replace these numbers"
                  n169 = call <vilib>:"WPI_PotentiometerGetNormalized.vi"("PotDevRef"=w256) -> ("Normalized Value"=w250:dbl)  [unwired: 8 in, 2 out]
                  n170 = global write "Robot Global Data.vi" "Collapse Arm Button"(TRUE ("Collapse Arm Button")) -> ()
                  n171 = global write "Robot Global Data.vi" "Extend Arm Button"(FALSE) -> ()
                  n172 = In Range and Coerce(upper limit=0.0 ("y"), x=w250, lower limit=-0.5) -> (In Range?=w249:bool)  [unwired: 1 out]
                  n173 = Wait (ms)(milliseconds to wait=u32 20) -> ()  [unwired: 1 out]
                }
              }
            }
          }
          frame True {
            n174 = flat-sequence {
              tunnel: w284 -> [w292]
              tunnel: [w290] -> w283
              tunnel: w282 -> [w290]
              tunnel: w281 -> [w291]
              tunnel: [w290] -> w279
              tunnel: w283 -> [w301]
              tunnel: w280 -> [w300]
              frame #0 {
                n175 = while {
                  tunnel: w292 -> [w298]
                  tunnel: w291 -> [w294]
                  stop <- w295 stop-if-true
                  # "replace these numbers"
                  n176 = call <vilib>:"WPI_PotentiometerGetNormalized.vi"("PotDevRef"=w298) -> ("Normalized Value"=w297:dbl)  [unwired: 8 in, 2 out]
                  n177 = call <vilib>:"WPI_MotorControlSetOutput.vi"("Output"=-0.5, "MotorControlDevRef"=w294) -> ()  [unwired: 7 in, 3 out]
                  n178 = Wait (ms)(milliseconds to wait=u32 40) -> ()  [unwired: 1 out]
                  n179 = Greater Or Equal?(x=w297, y=90.0) -> (x >= y?=w295:bool)
                }
              }
              frame #1 {
                n180 = while {
                  tunnel: w301 -> [w305]
                  tunnel: w300 -> [w303]
                  stop <- w304 stop-if-true
                  # "replace these numbers"
                  n181 = call <vilib>:"WPI_PotentiometerGetNormalized.vi"("PotDevRef"=w305) -> ("Normalized Value"=w307:dbl)  [unwired: 8 in, 2 out]
                  n182 = call <vilib>:"WPI_MotorControlSetOutput.vi"("Output"=-0.5, "MotorControlDevRef"=w303) -> ()  [unwired: 7 in, 3 out]
                  n183 = Greater Or Equal?(x=w307, y=90.0) -> (x >= y?=w304:bool)
                  n184 = Wait (ms)(milliseconds to wait=u32 40) -> ()  [unwired: 1 out]
                }
              }
            }
            n185 = while {
              tunnel: w279 -> [w286]
              stop <- w287 stop-if-true
              # "Extend"
              # "replace these numbers"
              n186 = call <vilib>:"WPI_PotentiometerGetNormalized.vi"("PotDevRef"=w286) -> ("Normalized Value"=w289:dbl)  [unwired: 8 in, 2 out]
              n187 = Greater Or Equal?(x=w289, y=90.0) -> (x >= y?=w287:bool)
              n188 = global write "Robot Global Data.vi" "Extend Arm Button"(TRUE) -> ()
            }
          }
        }
        n189 = Wait (ms)(milliseconds to wait=u32 100) -> ()  [unwired: 1 out]
      }
    }
    frame Enabled {
    }
  }
  n190 = disable-structure shown="Enabled" {
    frame Enabled {
      # "For probing values"
      n191 = global read "Robot Global Data.vi" "Pot Value Right"() -> (w315:dbl)
      n192 = global read "Robot Global Data.vi" "Pot Value"() -> (w316:dbl)
      n193 = call <vilib>:"WPI_AccelerometerRefNum Registry Get.vi"("refnum name"="accel") -> ("AccelerometerDevRef"=w320:T15)  [unwired: 9 in, 1 out]
      n194 = call <vilib>:"WPI_PotentiometerRefNum Registry Get.vi"("refnum name"="rightWheel") -> ("PotDevRef"=w313:T2)  [unwired: 9 in, 1 out]
      n195 = call <vilib>:"WPI_PotentiometerRefNum Registry Get.vi"("refnum name"="mechanismLeft") -> ("PotDevRef"=w311:T2)  [unwired: 9 in, 1 out]
      n196 = call <vilib>:"WPI_PotentiometerRefNum Registry Get.vi"("refnum name"="leftWheel") -> ("PotDevRef"=w312:T2)  [unwired: 9 in, 1 out]
      n197 = call <vilib>:"WPI_PotentiometerRefNum Registry Get.vi"("refnum name"="mechanismRight") -> ("PotDevRef"=w317:T2)  [unwired: 9 in, 1 out]
      n198 = call <vilib>:"WPI_GyroRefNum Registry Get.vi"("refnum name"="Gyro") -> ("GyroDevRef"=w309:T7)  [unwired: 9 in, 1 out]
      n199 = while {
        tunnel: w313 -> [w342]
        tunnel: w320 -> [w337]
        tunnel: w311 -> [w336]
        tunnel: w317 -> [w335]
        tunnel: w316 -> [w330]
        tunnel: w315 -> [w329]
        tunnel: w312 -> [w326]
        tunnel: w309 -> [w323]
        stop <- FALSE stop-if-true
        n200 = call <vilib>:"WPI_GyroGetAngle.vi"("GyroDevRef"=w323) -> ("Angle"=w324:dbl)  [unwired: 6 in, 4 out]
        n201 = call <vilib>:"WPI_AccelerometerGetAcceleration.vi"("AccelerometerDevRef"=w337) -> ("Accelerations"=w338:T21)  [unwired: 8 in, 2 out]
        n202 = call <vilib>:"WPI_PotentiometerGetNormalized.vi"("PotDevRef"=w342) -> ("Normalized Value"=w340:dbl)  [unwired: 8 in, 2 out]
        n203 = call <vilib>:"WPI_PotentiometerGetNormalized.vi"("PotDevRef"=w336) -> ("Normalized Value"=w334:dbl)  [unwired: 8 in, 2 out]
        n204 = call <vilib>:"WPI_PotentiometerGetNormalized.vi"("PotDevRef"=w326) -> ("Normalized Value"=w325:dbl)  [unwired: 8 in, 2 out]
        n205 = call <vilib>:"WPI_PotentiometerGetNormalized.vi"("PotDevRef"=w335) -> ("Normalized Value"=w332:dbl)  [unwired: 8 in, 2 out]
        n206 = Increment(x=w340) -> ()  [unwired: 1 out]
        n207 = Increment(x=w325) -> ()  [unwired: 1 out]
        n208 = disable-structure shown="Enabled" {
          disable-tunnel: w334 -> [w352 w357]
          disable-tunnel: [w353 w356] -> w333
          disable-tunnel: w330 -> [w351 _]
          frame Enabled {
            n209 = Subtract(x=w352, y=w351) -> (x-y=w355:dbl)
            n210 = Multiply(x=w355, y=-1505.88) -> (x*y=w353:dbl)
          }
          frame Disabled {
            n211 = expression code="-1505.88*(x-.587)"(w357) -> (w356:dbl)
          }
        }
        n212 = disable-structure shown="Enabled" {
          disable-tunnel: w332 -> [w346 w350]
          disable-tunnel: [w344 w349] -> w331
          disable-tunnel: w329 -> [w345 _]
          frame Enabled {
            n213 = Subtract(x=w346, y=w345) -> (x-y=w348:dbl)
            n214 = Multiply(x=w348, y=-1431.77) -> (x*y=w344:dbl)
          }
          frame Disabled {
            n215 = expression code="-1431.77*(x-0.961)"(w350) -> (w349:dbl)
          }
        }
        n216 = Unbundle By Name(w338) -> ("Y-Axis"=w328:dbl)
        n217 = Increment(x=w328) -> ()  [unwired: 1 out]
        n218 = call-poly <vilib>:"NT Write Value.vi"("Numeric"=w324, "Name"="Gyro") -> ()  [unwired: 9 in, 1 out]
        n219 = Increment(x=w331) -> ()  [unwired: 1 out]
        n220 = call-poly <vilib>:"NT Write Value.vi"("Numeric"=w333, "Name"="mechanismEncoder") -> ()  [unwired: 9 in, 1 out]
        n221 = Wait (ms)(milliseconds to wait=u32 150) -> ()  [unwired: 1 out]
      }
    }
    frame Disabled {
    }
  }
  n222 = disable-structure shown="Disabled" {
    frame Disabled {
      n223 = call <vilib>:"WPI_RobotDriveRefNum Registry Get.vi"("refnum name"="Drive 1") -> ("RobotDriveDevRef"=w358:T10)  [unwired: 9 in, 1 out]
      n224 = while {
        tunnel: w358 -> [w361]
        stop <- FALSE stop-if-true
        n225 = global read "Robot Global Data.vi" "Porticullis Tele"() -> (w360:bool)
        n226 = case shown="True" w360 {
          tunnel: w361 -> [_ w367]
          frame False {
            # "Nothing :)"
          }
          frame True {
            n227 = call "Set Arm Position.vi"("RobotDriveDevRef 2"=w367, "Setpoint"=100.0) -> ("RobotDriveDevRef"=w366:T10)  [unwired: 9 in]
            n228 = for {
              N: 40 -> [_]
              tunnel: w366 -> [w373]
              tunnel: [w373] -> w365
              n229 = Wait (ms)(milliseconds to wait=u32 50) -> ()  [unwired: 1 out]
            }
            n230 = for {
              N: 60 -> [_]
              tunnel: w365 -> [w371]
              tunnel: [w371] -> _
              n231 = call-poly <vilib>:"WPI_RobotDriveArcadeDrive.vi"("X axis value"=-0.5, "RobotDriveDevRef"=w371) -> ()  [unwired: 7 in, 3 out]
              n232 = Wait (ms)(milliseconds to wait=u32 50) -> ()  [unwired: 1 out]
            }
          }
        }
        n233 = Wait (ms)(milliseconds to wait=u32 200) -> ()  [unwired: 1 out]
      }
    }
    frame Enabled {
    }
  }
  n234 = disable-structure shown="Disabled" {
    frame Disabled {
      n235 = call <vilib>:"WPI_RobotDriveRefNum Registry Get.vi"("refnum name"="Drive 1") -> ("RobotDriveDevRef"=w375:T10)  [unwired: 9 in, 1 out]
      n236 = while {
        tunnel: w375 -> [w378]
        stop <- FALSE stop-if-true
        n237 = global read "Robot Global Data.vi" "CDF Tele"() -> (w377:bool)
        n238 = case shown="True" w377 {
          tunnel: w378 -> [_ w393]
          frame False {
            w381 = FALSE
            # "Nothing :)"
            n239 = global write "Robot Global Data.vi" "Arm Disable"(w381) -> ()
            n240 = global write "Robot Global Data.vi" "Drive Disable"(w381) -> ()
          }
          frame True {
            w384 = TRUE
            n241 = call <vilib>:"WPI_GyroRefNum Registry Get.vi"("refnum name"="Gyro") -> ("GyroDevRef"=w391:T7)  [unwired: 9 in, 1 out]
            n242 = global write "Robot Global Data.vi" "Arm Disable"(w384) -> ()
            n243 = global write "Robot Global Data.vi" "Drive Disable"(w384) -> ()
            n244 = call <vilib>:"WPI_GyroGetAngle.vi"("GyroDevRef"=w391) -> ("Angle"=w389:dbl)  [unwired: 6 in, 4 out]
            n245 = flat-sequence {
              tunnel: [w394] -> w383
              tunnel: w382 -> [_]
              frame #0 {
                n246 = global read "Robot Global Data.vi" "CDF Tele"() -> (w394:bool)
              }
            }
            n247 = call "Forward For inch.vi"("Angle robot facing"=w389, "Speed"=0.65, "Distance"=-13.0, "RobotDriveDevRef in"=w393) -> ("RobotDriveDevRef out"=w382:T10)  [unwired: 7 in]
            n248 = case shown="True" w383 {
              tunnel: w382 -> [w395 w397]
              tunnel: [w395 w396] -> w385
              frame False {
              }
              frame True {
                n249 = call "Set Arm Position.vi"("RobotDriveDevRef 2"=w397, "Speed"=0.9, "Setpoint"=620.0) -> ("RobotDriveDevRef"=w396:T10)  [unwired: 8 in]
                n250 = flat-sequence {
                  tunnel: w396 -> [_]
                  frame #0 {
                    "CDF Arm Down" <- TRUE
                  }
                }
              }
            }
            n251 = while {
              tunnel: w382 -> [w421]
              tunnel: [w420] -> _
              stop <- w416 stop-if-true
              n252 = local read "CDF Arm Down"() -> (w417:bool)
              n253 = global read "Robot Global Data.vi" "CDF Tele"() -> (w415:bool)
              n254 = call-poly <vilib>:"WPI_RobotDriveArcadeDrive.vi"("Y axis value"=-0.35, "X axis value"=0.0 ("Angle robot facing"), "RobotDriveDevRef"=w421) -> ("RobotDriveDevRef"=w420:T10)  [unwired: 6 in, 2 out]
              n255 = Wait (ms)(milliseconds to wait=u32 20) -> ()  [unwired: 1 out]
              n256 = Not(x=w415) -> (.not. x?=w414:bool)
              n257 = Or(x=w417, y=w414) -> (x .or. y?=w416:bool)
            }
            n258 = Tick Count (ms)() -> (millisecond timer value=w387:u32)
            n259 = while {
              tunnel: w385 -> [w412]
              tunnel: [w411] -> w386
              tunnel: w387 -> [w408]
              stop <- w403 stop-if-true
              n260 = global read "Robot Global Data.vi" "CDF Tele"() -> (w405:bool)
              n261 = call "Timeout.vi"("Start Time In"=w408, "Time Limit"=u32 2500) -> ("Timeout"=w404:bool)  [unwired: 8 in, 1 out]
              n262 = Not(x=w405) -> (.not. x?=w406:bool)
              n263 = call-poly <vilib>:"WPI_RobotDriveArcadeDrive.vi"("Y axis value"=-0.65, "X axis value"=0.0 ("Angle robot facing"), "RobotDriveDevRef"=w412) -> ("RobotDriveDevRef"=w411:T10)  [unwired: 6 in, 2 out]
              n264 = Or(x=w404, y=w406) -> (x .or. y?=w403:bool)
              n265 = Wait (ms)(milliseconds to wait=u32 20) -> ()  [unwired: 1 out]
            }
            n266 = while {
              tunnel: w386 -> [_]
              stop <- w401 stop-if-true
              n267 = global read "Robot Global Data.vi" "CDF Tele"() -> (w402:bool)
              n268 = Not(x=w402) -> (.not. x?=w401:bool)
            }
          }
        }
        n269 = Wait (ms)(milliseconds to wait=u32 200) -> ()  [unwired: 1 out]
      }
    }
    frame Enabled {
    }
  }
  n270 = disable-structure shown="Disabled" {
    frame Disabled {
      n271 = while {
        tunnel: i16[] [42, 16464, 3, 6, 16394, 376, 6, 16394, 377, 12, 16417, 1908, 24946, 26469, 29759, 2900, 24946, 26469, 29728, 17505, 29793] ("type string") -> [w424]
        stop <- FALSE stop-if-true
        # "put into PID loop"
        # "Get target information"
        # "if first false\n(target lost)"
        n272 = call-poly <vilib>:"NT Read Value.vi"("Name"="targetData") -> ("error out"=w440:errorcluster, "String"=w437:string)  [unwired: 9 in]
        n273 = Flattened String To Variant(4:w440, 6:w437, 7:w424) -> (0:w438:errorcluster, 3:w439:variant)
        n274 = Variant To Data(error in=w438, type=cluster{"x":dbl, "y":dbl, "target?":bool} {"x"=0.0, "y"=0.0, "target?"=FALSE} ("input cluster"), Variant=w439) -> (data=w433:cluster{"x":dbl, "y":dbl, "target?":bool})  [unwired: 1 out]
        n275 = Unbundle By Name(w433) -> ("target?"=w431:bool)
        n276 = feedback-in #5(w431) -> ()
        n277 = feedback #5(FALSE ("target?")) -> (w430:bool)
        n278 = Less?(x=w431, y=w430) -> (x < y?=w429:bool)
        n279 = feedback #6(cluster{"x out":dbl, "y out":dbl} {"x out"=10000.0, "y out"=0.0}) -> (w426:cluster{"x out":dbl, "y out":dbl})
        n280 = case shown="False" w431 {
          tunnel: w433 -> [_ w489]
          tunnel: [w443 w479] -> w432
          tunnel: w429 -> [w445 _]
          tunnel: [w442 w476] -> w427
          tunnel: w426 -> [w444 _]
          frame False {
            n281 = case shown="False" w445 {
              tunnel: w444 -> [w457 w475]
              tunnel: [w457 w465] -> w442
              tunnel: [w447 w461] -> w443
              frame False {
                # "no target"
                # "Angle to aim = \natan(targetY-robotY/targetX-Robotx)"
                n282 = global read "Robot Global Data.vi" "poses"() -> (w451:cluster{"theta":dbl}[])
                n283 = Index Array(array=w451, index=0) -> (element=w450:cluster{"theta":dbl})
                n284 = Unbundle By Name(w450) -> ("x"=w455:dbl, "y"=w453:dbl)
                n285 = Unbundle(w457) -> ("x out"=w456:dbl, "y out"=w454:dbl)
                n286 = Subtract(x=w456, y=w455) -> (x-y=w448:dbl)
                n287 = Subtract(x=w454, y=w453) -> (x-y=w449:dbl)
                n288 = Inverse Tangent (2 Input)(1:w448, 2:w449) -> (0:w446:dbl)
                n289 = expression code="(x/pi)*180.0" ("radians to degrees")(w446) -> (w447:dbl)
              }
              frame True {
                # "no target"
                # "last target\nlocation"
                # "pose when target last seen"
                # "Find target in field space"
                # "translate by \nrobot location"
                # "rotate by\ngyro angle"
                n290 = global read "Robot Global Data.vi" "poses"() -> (w463:cluster{"theta":dbl}[])
                n291 = Unbundle(w475) -> ("x out"=w459:dbl, "y out"=w458:dbl)
                n292 = Index Array(array=w463, index=19) -> (element=w462:cluster{"theta":dbl})
                n293 = Unbundle(w462) -> (w470:dbl, w469, w468)
                n294 = expression code="(x/180.0)*pi" ("degrees to radians")(w470) -> (w474:dbl)
                n295 = call-poly <vilib>:"2D Cartesian Coordinate Rotation.vi"("theta"=w474, "y"=w458, "x"=w459) -> ("y out"=w472:dbl, "x out"=w473:dbl)  [unwired: 6 in, 1 out]
                n296 = Bundle(w469, w468) -> (w471:cluster{void, void})  [unwired: 1 in]
                n297 = call-poly <vilib>:"2D Cartesian Coordinate Shift.vi"("shift"=w471, "Y"=w472, "X"=w473) -> ("Y Out"=w466:dbl[], "X Out"=w467:dbl[])  [unwired: 6 in, 1 out]
                n298 = Bundle("X Out"=w467, "Y Out"=w466) -> (w465:cluster{"X Out":dbl[], "Y Out":dbl[]})  [unwired: 1 in]
                n299 = Inverse Tangent (2 Input)(1:w459, 2:w458) -> (0:w460:dbl)
                n300 = expression code="(x/pi)*180.0" ("radians to degrees")(w460) -> (w461:dbl)
              }
            }
          }
          frame True {
            # "last seen target"
            # "target visible"
            # "find angle to turn to"
            # "At time picture was taken"
            # "Find angle"
            # "camera offset\n(left + towards rear = positive)"
            n301 = Unbundle By Name(w489) -> ("x"=w488:dbl, "y"=w487:dbl)
            n302 = call-poly <vilib>:"2D Cartesian Coordinate Shift.vi"("shift"=cluster{"dx":dbl, "dy":dbl} {"dx"=0.0, "dy"=0.0}, "y"=w487, "x"=w488) -> ("y out"=w477:dbl, "x out"=w478:dbl)  [unwired: 6 in, 1 out]
            n303 = Inverse Tangent (2 Input)(1:w478, 2:w477) -> (0:w485:dbl)
            n304 = Bundle("x out"=w478, "y out"=w477) -> (w476:cluster{"x out":dbl, "y out":dbl})  [unwired: 1 in]
            n305 = expression code="(x/pi)*180.0" ("radians to degrees")(w485) -> (w484:dbl)
            n306 = global read "Robot Global Data.vi" "poses"() -> (w483:cluster{"theta":dbl}[])
            n307 = Index Array(array=w483, index=19) -> (element=w481:cluster{"theta":dbl})
            n308 = Unbundle By Name(w481) -> ("theta"=w480:dbl)
            n309 = Add(x=w484, y=w480) -> (x+y=w479:dbl)
          }
        }
        n310 = feedback-in #6(w427) -> ()
        n311 = global write "Robot Global Data.vi" "Target Heading"(w432) -> ()
        n312 = Wait (ms)(milliseconds to wait=u32 20) -> ()  [unwired: 1 out]
      }
    }
    frame Enabled {
    }
  }
  n313 = disable-structure shown="Disabled" {
    frame Disabled {
      # "because sometimes the velocity appears to dip to 0 even if the arm is moving, why not add this\nto make sure it is 0 for a period of 100 ms"
      n314 = Less?(y=0.8) -> (x < y?=w493:bool)  [unwired: 1 in]
      n315 = feedback #7(0.0 ("angle B 2")) -> (w492:dbl)
      n316 = case shown="True" w493 {
        tunnel: [0.0 w498] -> w491
        tunnel: w492 -> [_ w497]
        frame False {
        }
        frame True {
          n317 = Increment(x=w497) -> (x+1=w498:dbl)
        }
      }
      n318 = feedback-in #7(w491) -> ()
      n319 = Greater Or Equal?(x=w491, y=5.0) -> ()  [unwired: 1 out]
    }
    frame Enabled {
    }
  }
  n320 = disable-structure shown="Disabled" {
    frame Disabled {
      n321 = while {
        stop <- FALSE stop-if-true
        n322 = global read "Robot Global Data.vi" "Automated Aim"() -> (w500:bool)
        n323 = Wait (ms)(milliseconds to wait=u32 200) -> ()  [unwired: 1 out]
        n324 = case shown="True" w500 {
          frame False {
          }
          frame True {
            n325 = call <vilib>:"WPI_RobotDriveRefNum Registry Get.vi"("refnum name"="Drive 1") -> ("RobotDriveDevRef"=w502:T10)  [unwired: 9 in, 1 out]
            n326 = while {
              tunnel: w502 -> [w506]
              stop <- w510 stop-if-true
              n327 = call-poly <vilib>:"NT Read Value.vi"("Name"="xPosition") -> ("Numeric"=w505:dbl)  [unwired: 9 in, 1 out]
              n328 = Subtract(x=w505, y=85.0) -> (x-y=w515:dbl)
              n329 = Not Equal To 0?(x=w505) -> (x != 0?=w504:bool)
              n330 = Divide(x=w515, y=80.0) -> (x/y=w513:dbl)
              n331 = call-poly <vilib>:"PID.vi"("output range"=cluster{"output high":dbl, "output low":dbl} {"output high"=0.6, "output low"=-0.6}, "PID gains"=T14 {"proportional gain (Kc)"=5.0, "integral time (Ti, min)"=0.03, "derivative time (Td, min)"=0.03} ("Turn robot to camera 2"), "process variable"=w513, "setpoint"=0.0) -> ("output"=w519:dbl)  [unwired: 6 in, 1 out]
              n332 = global read "Robot Global Data.vi" "Automated Aim"() -> (w511:bool)
              n333 = Negate(x=w519) -> (-x=w509:dbl)
              n334 = Select(t=w509, s=w504, f=0.0) -> (s? t:f=w507:dbl)
              n335 = Wait (ms)(milliseconds to wait=u32 20) -> ()  [unwired: 1 out]
              n336 = call-poly <vilib>:"WPI_RobotDriveArcadeDrive.vi"("X axis value"=w507, "RobotDriveDevRef"=w506) -> ()  [unwired: 7 in, 3 out]
              n337 = Not(x=w511) -> (.not. x?=w510:bool)
            }
          }
        }
      }
    }
    frame Enabled {
    }
  }
  n338 = disable-structure shown="Disabled" {
    frame Disabled {
      n339 = for {
        N: 4 -> [_]
        n340 = for {
          N: 3 -> [_]
          tunnel: _ -> [w527]
          tunnel: [w528] -> w525
          n341 = call <vilib>:"WPI_MotorControlSetOutput.vi"("Output"=-0.35 ("Left axis value"), "MotorControlDevRef"=w527) -> ("MotorControlDevRef"=w528:T11)  [unwired: 7 in, 2 out]
          n342 = Wait (ms)(milliseconds to wait=u32 50) -> ()  [unwired: 1 out]
        }
        n343 = for {
          N: 3 -> [_]
          tunnel: w525 -> [w531]
          tunnel: [w532] -> _
          n344 = call <vilib>:"WPI_MotorControlSetOutput.vi"("Output"=0.35 ("Left axis value"), "MotorControlDevRef"=w531) -> ("MotorControlDevRef"=w532:T11)  [unwired: 7 in, 2 out]
          n345 = Wait (ms)(milliseconds to wait=u32 50) -> ()  [unwired: 1 out]
        }
      }
    }
    frame Enabled {
    }
  }
  n346 = disable-structure shown="Enabled" {
    frame Enabled {
      n347 = Random Number (0-1)() -> (number: 0 to 1=w537:dbl)
      n348 = Format Into String(format string="/home/lvuser/data-%.6f.csv", w537) -> (resulting string=w535:string)  [unwired: 2 in, 1 out]
      n349 = String To Path(string=w535) -> (path=w534:path)
      n350 = Open/Create/Replace File(file path (use dialog)=w534, operation (0:open)=T22."replace or create", access (0:read/write)=enum16{"read/write", "read-only", "write-only"}."write-only") -> (refnum out=w542:refnum<file>, error out=w539:errorcluster)  [unwired: 3 in, 1 out]
      n351 = while {
        tunnel: w542 -> [w566]
        tunnel: [w553] -> w541
        tunnel: w539 -> [w548]
        tunnel: [w544] -> w538
        i -> [w564]
        stop <- FALSE stop-if-true
        w565 = u32 50 ("milliseconds to wait")
        # "This while loop can be used \nif other data needs to be written. \nDisabled for now because we don't need to write \nany other data."
        n352 = Wait (ms)(milliseconds to wait=w565) -> ()  [unwired: 1 out]
        n353 = Multiply(x=w565, y=w564) -> (x*y=w563:u32)
        n354 = call <vilib>:"WPI_Power Get PDP Currents.vi"() -> ("all currents (A)"=w552:dbl[])  [unwired: 13 in, 2 out]
        n355 = call <vilib>:"WPI_Power Get PDP Voltage.vi"() -> ("voltage (V)"=w557:dbl)  [unwired: 14 in, 1 out]
        n356 = Number To Decimal String(number=w563) -> (decimal integer string=w562:string)  [unwired: 1 in]
        n357 = Write to Text File(file (use dialog)=w566, text=w562, error in=w548) -> (refnum out=w561:refnum<file>, error out=w547:errorcluster)  [unwired: 1 in, 1 out]
        n358 = Write to Text File(file (use dialog)=w561, text=",", error in=w547) -> (refnum out=w560:refnum<file>, error out=w546:errorcluster)  [unwired: 1 in, 1 out]
        n359 = Build Array (concatenate)(w552, w557) -> (w556:dbl[])
        n360 = for {
          tunnel: w560 -> [w580]
          tunnel: [w574] -> w558
          tunnel: w556 -> [w573] mode=indexing
          tunnel: w546 -> [w572]
          tunnel: [w571] -> w545
          n361 = Format Into String(format string="%f", w573) -> (resulting string=w578:string)  [unwired: 2 in, 1 out]
          n362 = Write to Text File(file (use dialog)=w580, text=w578, error in=w572) -> (refnum out=w576:refnum<file>, error out=w577:errorcluster)  [unwired: 1 in, 1 out]
          n363 = Write to Text File(file (use dialog)=w576, text=",", error in=w577) -> (refnum out=w574:refnum<file>, error out=w571:errorcluster)  [unwired: 1 in, 1 out]
        }
        n364 = disable-structure shown="Enabled" {
          disable-tunnel: w558 -> [w569 w570]
          disable-tunnel: [w567 w570] -> w554
          frame Disabled {
            n365 = for {
              n366 = Write to Text File() -> ()  [unwired: 4 in, 3 out]
            }
            n367 = Write to Text File(file (use dialog)=w569, text="\n") -> (refnum out=w567:refnum<file>)  [unwired: 2 in, 2 out]
          }
          frame Enabled {
          }
        }
        n368 = Concatenate Strings("\r", "\n") -> (w549:string)
        n369 = Write to Text File(file (use dialog)=w554, text=w549, error in=w545) -> (refnum out=w553:refnum<file>, error out=w544:errorcluster)  [unwired: 1 in, 1 out]
      }
      n370 = Close File(refnum=w541, error in=w538) -> ()  [unwired: 2 out]
    }
    frame Disabled {
    }
  }
  "error out (no error)" <- "error in (no error)"
